vi "Globaltracker.vi"() -> ()   [LabVIEW 2016]
uses:
  <vilib>/picture/picture.llb/imagedata.ctl
panel:
  out "Cage orientation swapped":bool
  in  "index":i16
  in  "CounterUpforPlaybackSpeed":i16
  in  "CounterDownforPlaybackSpeed":i16
  in  "KeyboardShortCuts":string[][](array[string])
  out "Defaultsettings":bool
  out "fulltrackbackgroundregions":u32[][](array[numeric]) format="%x"
  out "fulltrackbackground":u32[][](array[numeric]) format="%x"
  out "TrackerDisabled":bool
  in  "Progressbar":u16
  in  "K":dbl
  out "Kalmanfilter":bool
  out "NoFilter":bool
  out "Analysiss":bool
  out "loadedregions":u32[][](array[numeric]) format="%x"
  out "mousepixmap":u32[][](array[numeric]) format="%x"
  out "MouseImage":T1
  out "TTLFuncionEnable":bool
  out "Region(TTL)":i32
  out "Done":bool
  out "TTL":T2(array[cluster])
  out "TTLSignalActive":bool
  out "Colors":u32[](array[numeric])
  out "SegmentsInMatrix":u32[][](array[numeric])
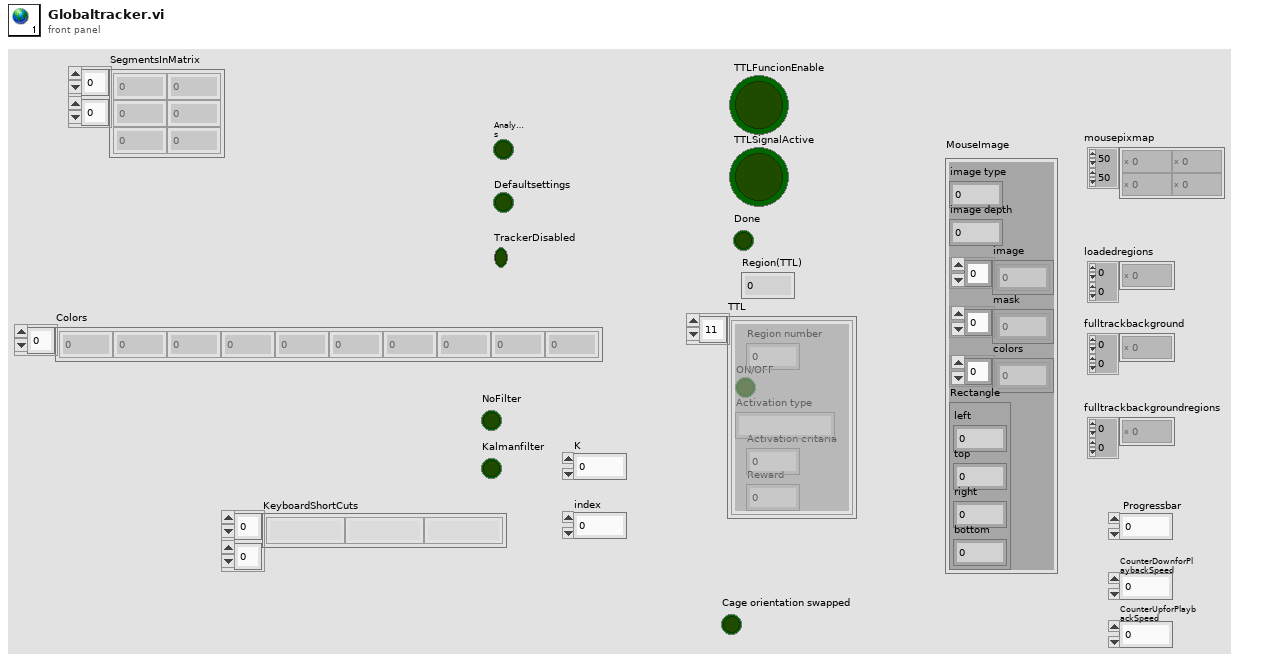
[diagram p1: front panel]
types:
  T1 = typedef "imagedata.ctl" = cluster{"image type":i32, "image depth":i32, "image":u8[], "mask":u8[], "colors":u32[], "Rectangle":cluster{"left":i16, "top":i16, "right":i16, "bottom":i16}}
  T2 = cluster{"Region number":i32, "ON/OFF":bool, "Activation type":string, "Activation critaria":i32, "Reward":i32}[]
diagram:
